vi "To JSON String.vi"(0 "Display State In":T1, 5 "enable LabVIEW extensions? (T)":bool=TRUE, 7 "pretty print? (F)":bool, 9 "Container State":T2, 11 "error in (no error)":errorcluster) -> (4 "Display State Out":T1, 8 "JSON String":string, 15 "error out":errorcluster)   [LabVIEW 2017, in "Variant Tree API.lvlib" / "Variant Tree.xctl"]
uses:
  Variant Tree.xctl
  <vilib>/_xctls/Container State.ctl
  State.ctl
  <vilib>/National Instruments/Variant JSON API/Variant JSON API.lvlib
  <vilib>/_xctls/XControlSupport.lvlib
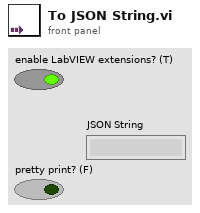
[diagram p1: front panel]
types:
  T1 = typedef "Variant Tree API.lvlib/Variant Tree.xctl/State.ctl" = cluster{"Numeric":dbl}
  T2 = typedef "XControlSupport.lvlib/Container State.ctl" = cluster{"Indicator?":bool, "Run Mode?":bool, " Refnum":refnum<vi>}
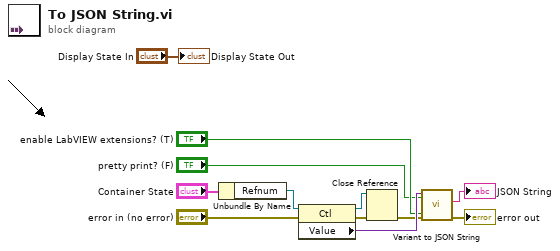
[diagram p0: block diagram]
diagram:
  n1 = Unbundle By Name("Container State") -> ("Refnum"=w10:refnum<vi>)
  n2 = property class="Ctl"(reference=w10, error in="error in (no error)") -> (reference out=w1:refnum<vi>, error out=w7:errorcluster, "Value"=w9:variant)
  n3 = Close Reference(reference=w1, error in (no error)=w7) -> (error out=w2:errorcluster)
  n4 = call <vilib>:"Variant to JSON String.vi"("enable LabVIEW extensions? (T)"="enable LabVIEW extensions? (T)", "pretty print? (F)"="pretty print? (F)", "error in (no error)"=w2, "Variant in"=w9) -> ("error out"=→"error out":errorcluster, "String"=→"JSON String":string)  [unwired: 5 in, 1 out]
  "Display State Out" <- "Display State In"
